vi "Set Readout Rate.vi"(8 "error in (no error)":errorcluster, 11 "CCDCamera in":refnum<class "Real Camera.lvclass">) -> (0 "error out":errorcluster, 3 "CCDCamera out":refnum<class "Real Camera.lvclass">)   [LabVIEW 2018, in "Real Camera.lvclass"]
doc: "Set readout rate"
uses:
  Real Camera.lvclass
  C:/Users/Denis/Desktop/S4ACS/S4ACS/Simulated_CCD_Camera/Simulated Camera.lvclass
  Simulated_CCD_Camera/Simulated Camera.lvclass
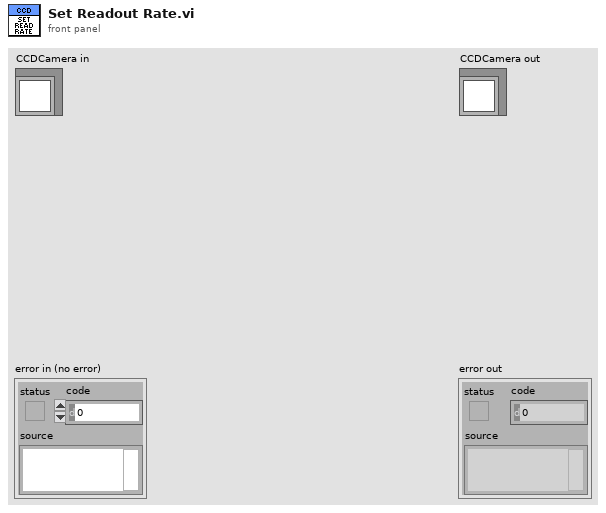
[diagram p1: front panel]
types:
  T1 = cluster{"PREAMP":u16, "READOUT_RATE":u16, "EM_GAIN":u16, "VERTICAL_SHIFT_SPEED":u16, "READ_MODE":u16, "FRAME_TRANSFER":bool, "VERTICAL_CLOCK_VOLTAGE":u16, "ACQUISITION_MODE":u16, "AD_CHANNEL":u16, "EM_MODE":u16, "SHUTTER_TTL":u16, "SHUTTER_OPENING_TIME":u16, "SHUTTER_CLOSING_TIME":u16, "SHUTTER_MODE":u16, "TRIGGER_MODE":u16, "VBIN":u16, "INITIAL_LINE":u16, "INITIAL_COLUMN":u16, "FINAL_LINE":u16, "FINAL_COLUMN":u16, "HBIN":u16}
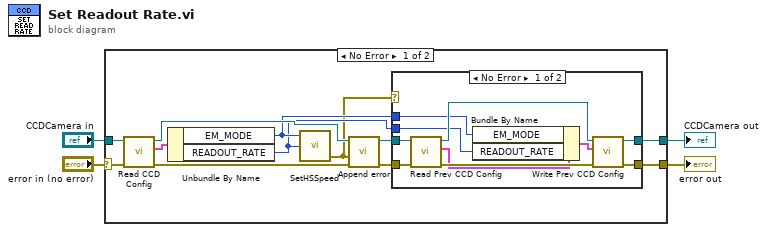
[diagram p0: block diagram]
diagram:
  n1 = case shown="No Error" "error in (no error)" {
    selector: "error in (no error)" -> [w16 w30]
    tunnel: [w6 w30] -> w4
    tunnel: [w7 w29] -> w3
    tunnel: "CCDCamera in" -> [w14 w29]
    frame No Error {
      n2 = call "Read CCD Config.vi"("error in (no error)"=w16, "CCDCamera in"=w14) -> ("error out"=w13:errorcluster, "CCD Config"=w15:T1, "CCDCamera out"=w12:refnum<class "Real Camera.lvclass">)  [unwired: 7 in]
      n3 = Unbundle By Name(w15) -> ("EM_MODE"=w11:u16, "READOUT_RATE"=w10:u16)
      n4 = call <userlib>:"SetHSSpeed.vi"("index"=w10, "type"=w11) -> ("error out"=w5:errorcluster)  [unwired: 2 in, 1 out]
      n5 = call "Append error.vi"("error in (no error)"=w13, "error"=w5, "Simulated_CCD_Camera in"=w12) -> ("error out"=w9:errorcluster, "Simulated_CCD_Camera out"=w8:refnum<class "Real Camera.lvclass">)  [unwired: 7 in]
      n6 = case shown="No Error" w5 {
        tunnel: [w25 w28] -> w7
        tunnel: [w23 w27] -> w6
        tunnel: w11 -> [w20 _]
        tunnel: w10 -> [w19 _]
        tunnel: w9 -> [w18 w27]
        tunnel: w8 -> [w17 w28]
        frame No Error {
          n7 = call-dynamic "Read Prev CCD Config.vi"("error in (no error)"=w18, "Simulated_CCD_Camera in"=w17) -> ("error out"=w24:errorcluster, "Prev CCD Config"=w22:T1, "Simulated_CCD_Camera out"=w26:refnum<class "Real Camera.lvclass">)  [unwired: 7 in]
          n8 = Bundle By Name(cluster=w22, "EM_MODE"=w20, "READOUT_RATE"=w19) -> (w21:T1)
          n9 = call-dynamic "Write Prev CCD Config.vi"("error in (no error)"=w24, "Prev CCD Config"=w21, "Simulated_CCD_Camera in"=w26) -> ("error out"=w23:errorcluster, "Simulated_CCD_Camera out"=w25:refnum<class "Real Camera.lvclass">)  [unwired: 7 in]
        }
        frame Error {
        }
      }
    }
    frame Error {
    }
  }
  "error out" <- w4
  "CCDCamera out" <- w3
